vi "Read Coords.vi"(8 "error in (no error)":errorcluster, 11 "ControlDragStartingMsg In":refnum<class "ControlDragStartingMsg.lvclass">) -> (0 "error out":errorcluster, 2 "Coords":T1, 3 "ControlDragStartingMsg Out":refnum<class "ControlDragStartingMsg.lvclass">)   [LabVIEW 2020, in "MVA Framework.lvlib" / "ActorEvents.lvlib" / "ControlDragStartingMsg.lvclass"]
uses:
  ControlDragStartingMsg.lvclass
  <vilib>/Utility/miscctls.llb/LVPoint32TypeDef.ctl
  ControlDragStartingMsg.lvclass/ControlDragStartingMsg.ctl
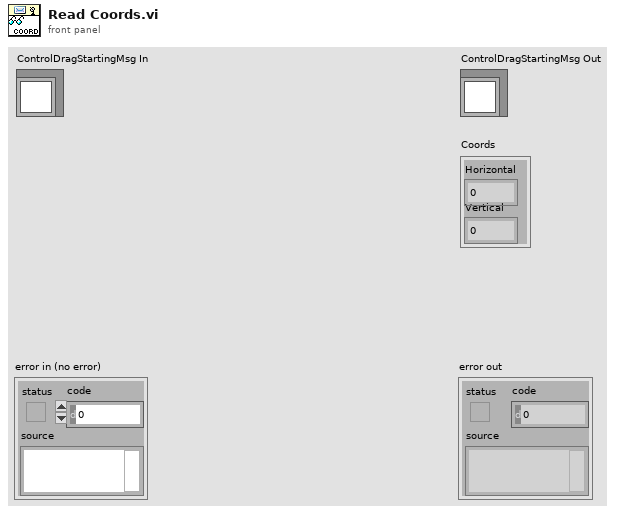
[diagram p1: front panel]
types:
  T1 = typedef "LVPoint32TypeDef.ctl" = cluster{"Horizontal":i32, "Vertical":i32}
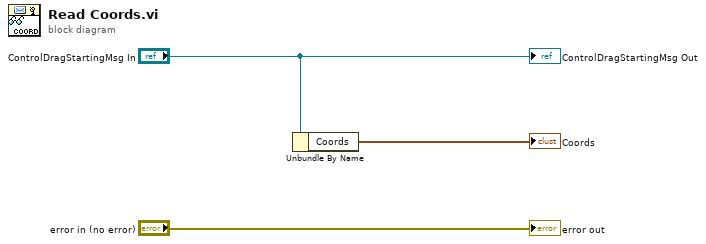
[diagram p0: block diagram]
diagram:
  n1 = Unbundle By Name("ControlDragStartingMsg In") -> ("Coords"=→"Coords":T1)
  "error out" <- "error in (no error)"
  "ControlDragStartingMsg Out" <- "ControlDragStartingMsg In"
